vi "Value Change.vi"(7 "objects":T1, 8 "error in":errorcluster, 11 "Table Manager in":refnum<class "Table Manager.lvclass">) -> (0 "error out":errorcluster, 2 "Update?":bool, 3 "Table Manager out":refnum<class "Table Manager.lvclass">)   [LabVIEW 2014, in "Table Manager.lvlib" / "Table Manager.lvclass"]
uses:
  Table Manager.lvclass
  object ref.ctl
  Configuration Editor/Classes/Engine Parent/Engine Parent Editor Node.lvclass
  Configuration Editor/Classes/Module editor node/module editor node.lvclass
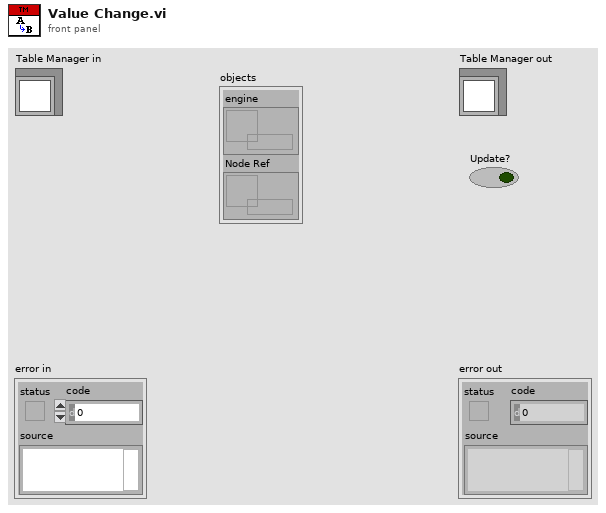
[diagram p1: front panel]
types:
  T1 = typedef "Table Manager.lvlib/Table Manager.lvclass/object ref.ctl" = cluster{"engine":refnum<data-value>, "Node Ref":refnum<data-value>}
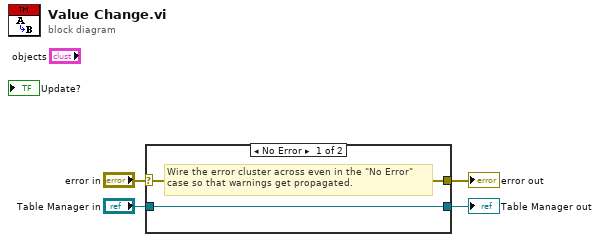
[diagram p0: block diagram]
diagram:
  n1 = case shown="No Error" "error in" {
    selector: "error in" -> [w5 w8]
    tunnel: [w5 w8] -> w3
    tunnel: [w6 w7] -> w1
    tunnel: "Table Manager in" -> [w6 w7]
    frame No Error {
      # "Wire the error cluster across even in the \"No Error\"\ncase so that warnings get propagated."
    }
    frame Error {
    }
  }
  "error out" <- w3
  "Table Manager out" <- w1
